vi "Is Defined.vi"(11 "Value in":refnum<class "Value.lvclass">) -> (2 "Is Defined?":bool, 3 "Value out":refnum<class "Value.lvclass">)   [LabVIEW 2024, in "Electronic Datasheet.lvlib" / "Value.lvclass"]
uses:
  Value.lvclass
  Value.lvclass/Value.ctl
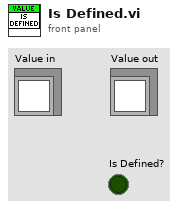
[diagram p1: front panel]
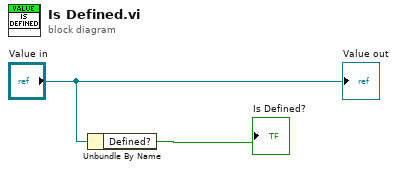
[diagram p0: block diagram]
diagram:
  n1 = Unbundle By Name("Value in") -> ("Defined?"=→"Is Defined?":bool)
  "Value out" <- "Value in"
